vi "DCA Get Limit Data From Run Data.vi"(7 "Limit":T1, 8 "error in (no error)":errorcluster, 10 "Run Waveforms":waveform(dbl)[](array[waveform]), 11 "File Information":T6) -> (0 "error out":errorcluster, 1 "Data Waveform":waveform(dbl), 3 "Found?":bool)   [LabVIEW 2011]
uses:
  server/TDMS/TDMS File.ctl
  server/TDMS/TDMS Run.ctl
  server/TDMS/TDMS Channel (Sxx).ctl
  server/database/Fields/Field Record.ctl
  server/database/Fields/Field DataTypes.ctl
  server/database/Fields/Field NextItem.ctl
  TypeDefs/DCA Limit.ctl
  TypeDefs/DCA Limit Quantity.ctl
  TypeDefs/DCA Limit Comparison.ctl
  TypeDefs/DCA Limit Operation.ctl
  Test Referential Limit.ctl
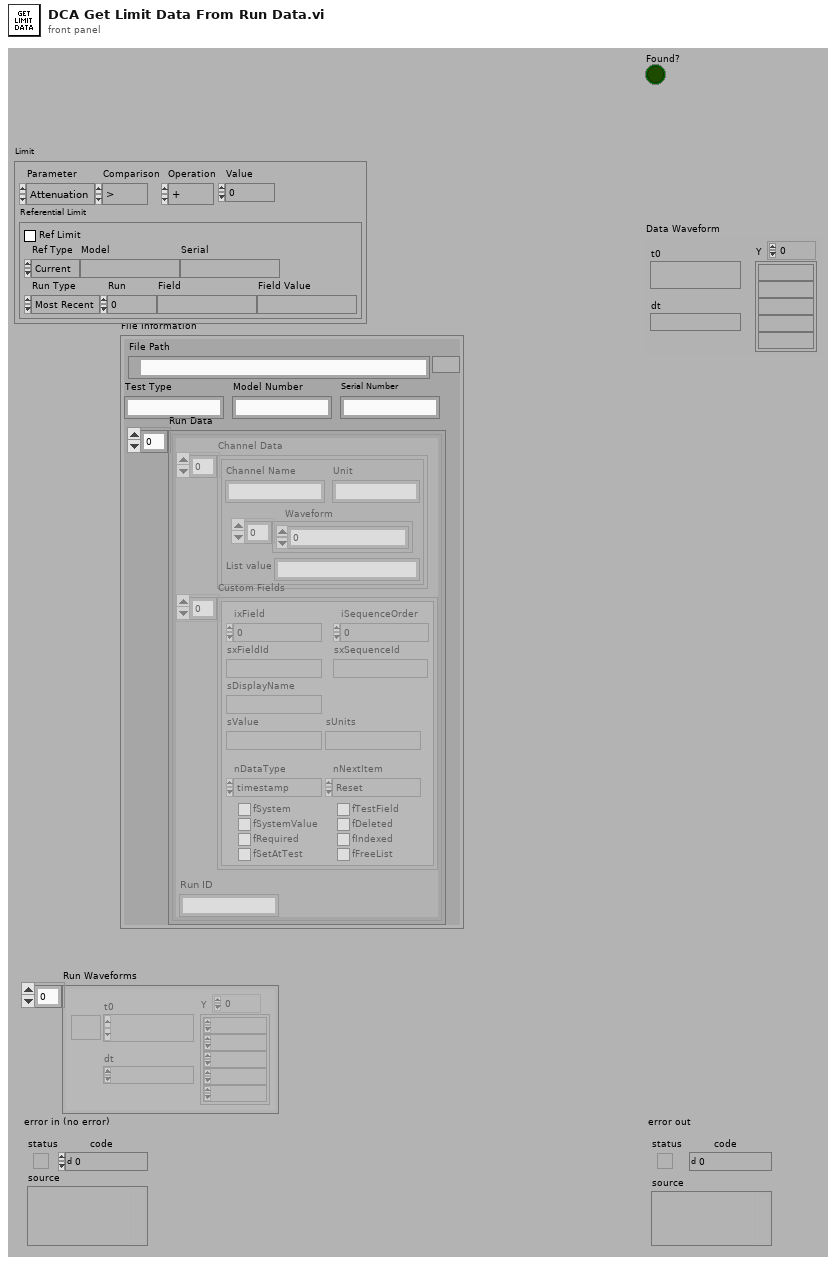
[diagram p1: front panel]
types:
  T1 = typedef "DCA Limit.ctl" = cluster{"Parameter":T2, "Comparison":T3, "Operation":T4, "Value":dbl, "Referential Limit":T5}
  T2 = typedef "DCA Limit Quantity.ctl" = enum16{"Attenuation", "Zin", "Zout", "R1", "R2", "R3", "Rab", "Rac", "Rbc"}
  T3 = typedef "DCA Limit Comparison.ctl" = enum16{">", ">=", "<", "<="}
  T4 = typedef "DCA Limit Operation.ctl" = enum16{"+", "-"}
  T5 = typedef "Test Referential Limit.ctl" = cluster{"Ref Limit":bool, "Ref Type":enum16{"Current", "Specify"}, "Model":string, "Serial":string, "Run Type":enum16{"Most Recent", "Run #", "Match Field"}, "Run":i32, "Field":string, "Field Value":string}
  T6 = typedef "TDMS File.ctl" = cluster{"File Path":path, "Run Data":T7[], "Serial Number":string, "Model Number":string, "Test Type":string}
  T7 = typedef "TDMS Run.ctl" = cluster{"Channel Data":T8[], "Custom Fields":T9[], "Run ID":string}
  T8 = typedef "TDMS Channel (Sxx).ctl" = cluster{"Channel Name":string, "Waveform":dbl[], "Unit":string, "List value":string}
  T9 = typedef "Field Record.ctl" = cluster{"ixField":i32, "iSequenceOrder":i32, "sxFieldId":string, "sxSequenceId":string, "sDisplayName":string, "sValue":string, "sUnits":string, "nDataType":T10, "nNextItem":T11, "fSystem":bool, "fSystemValue":bool, "fRequired":bool, "fSetAtTest":bool, "fTestField":bool, "fDeleted":bool, "fIndexed":bool, "fFreeList":bool}
  T10 = typedef "Field DataTypes.ctl" = enum32{"text", "numeric", "list", "timestamp", "boolean"}
  T11 = typedef "Field NextItem.ctl" = enum32{"Reset", "Retain", "Auto-Increment"}
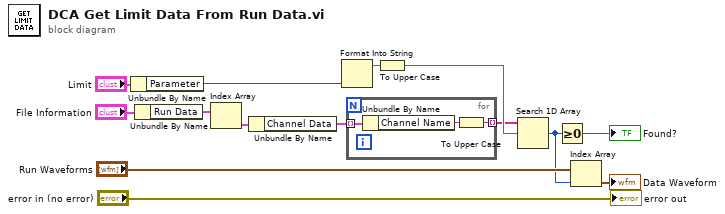
[diagram p0: block diagram]
diagram:
  n1 = Unbundle By Name("Limit") -> ("Parameter"=w2:T2)
  n2 = Unbundle By Name("File Information") -> ("Run Data"=w10:T7[])
  n3 = Index Array(array=w10) -> (element=w11:T7)  [unwired: 1 in]
  n4 = Unbundle By Name(w11) -> ("Channel Data"=w8:T8[])
  n5 = Format Into String(w2) -> (resulting string=w12:string)  [unwired: 3 in, 1 out]
  n6 = for {
    tunnel: w8 -> [w17] mode=indexing
    tunnel: [w15] -> w6 mode=indexing
    n7 = Unbundle By Name(w17) -> ("Channel Name"=w16:string)
    n8 = To Upper Case(1:w16) -> (0:w15:string)
  }
  n9 = To Upper Case(1:w12) -> (0:w7:string)
  n10 = Search 1D Array(1D array=w6, element=w7) -> (index of element=w3:i32)  [unwired: 1 out]
  n11 = Greater Or Equal To 0?(x=w3) -> (x >= 0?=→"Found?":bool)
  n12 = Index Array(array="Run Waveforms", index=w3) -> (element=→"Data Waveform":waveform(dbl))
  "error out" <- "error in (no error)"
